vi "Add Bus Monitor.vi"(8 "error in":errorcluster, 10 "new busMonitor":refnum<k24>, 11 "1553channel ref in":refnum<k24>) -> (0 "error out":errorcluster, 3 "1553channel ref out":refnum<k24>)   [LabVIEW 2020, in "Ballard_1553_Hardware_ni.lvlib"]
uses:
  Ballard_1553_Hardware_ni.lvlib
  C:/Users/Administrator/Desktop/GIT/Ballard-MIL-STD-1553-Custom-Device/Source/System Explorer/SubVIs/Parse XML Ballard/1.2/BTIXML_SerDes.dll
  Ballard-MIL-STD-1553-Custom-Device/Source/System Explorer/SubVIs/Parse XML Ballard/1.2/BTIXML_SerDes.dll
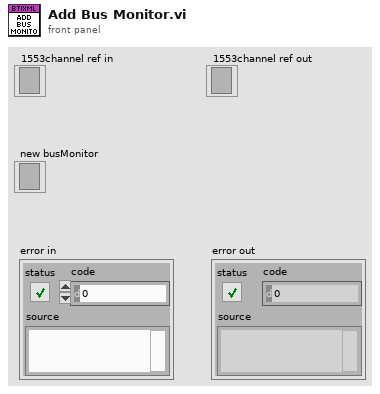
[diagram p1: front panel]
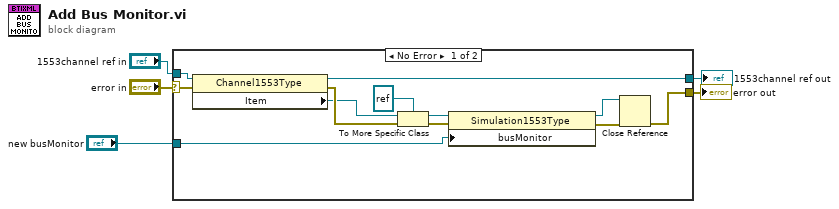
[diagram p0: block diagram]
diagram:
  n1 = case shown="No Error" "error in" {
    selector: "error in" -> [w15 w18]
    tunnel: [w6 w18] -> w5
    tunnel: [w17 w19] -> w4
    tunnel: "1553channel ref in" -> [w16 w19]
    tunnel: "new busMonitor" -> [w9 _]
    frame No Error {
      n2 = property class="Channel1553Type"(reference=w16, error in=w15) -> (reference out=w17:refnum<k24>, error out=w14:errorcluster, "Item"=w13:refnum<k24>)
      n3 = To More Specific Class(target class=refnum<k24> refnum, reference=w13, error in=w14) -> (specific class reference=w11:refnum<k24>, error out=w10:errorcluster)
      n4 = property class="Simulation1553Type"(reference=w11, error in=w10, "busMonitor"=w9) -> (reference out=w7:refnum<k24>, error out=w8:errorcluster)
      n5 = Close Reference(reference=w7, error in (no error)=w8) -> (error out=w6:errorcluster)
    }
    frame Error {
    }
  }
  "error out" <- w5
  "1553channel ref out" <- w4
